vi "Exp.vi"() -> ()   [LabVIEW 2015]
panel:
  out "Error Out":errorcluster
  in  "Error In":errorcluster
  in  "Stop Button":bool
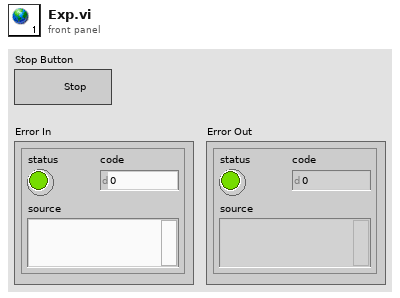
[diagram p1: front panel]
diagram:
